vi "Process input and Make Stacks.vi"(11 "input":string[](array[string])) -> (2 "Moves":string[](array[string]), 3 "Stacks":cluster{"Label":string, "Stack":string[]}[](array[cluster]))   [LabVIEW 2021]
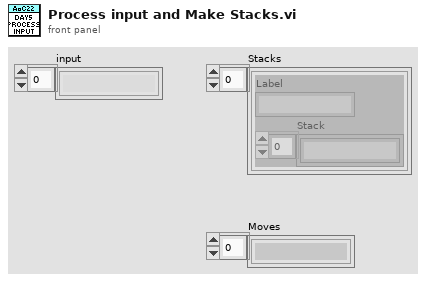
[diagram p1: front panel]
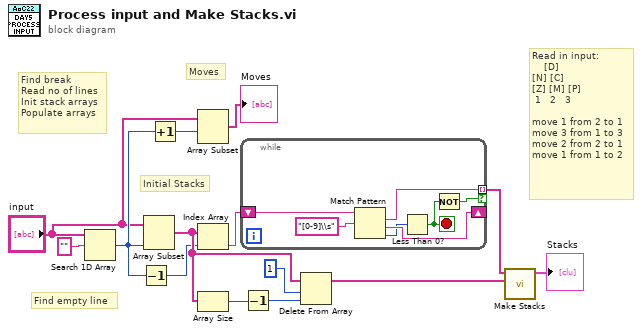
[diagram p0: block diagram]
diagram:
  # "Initial Stacks"
  # "Moves"
  # "Find empty line"
  # "Find break\nRead no of lines\nInit stack arrays\nPopulate arrays"
  # "Read in input:\n    [D]    \n[N] [C]    \n[Z] [M] [P]\n 1   2   3 \n\nmove 1 from 2 to 1\nmove 3 from 1 to 3\nmove 2 from 2 to 1\nmove 1 from 1 to 2"
  n1 = Search 1D Array(1D array="input", element="") -> (index of element=w11:i32)  [unwired: 1 in]
  n2 = Decrement(x=w11) -> (x-1=w5:i32)
  n3 = Array Subset(array="input", length=w11) -> (w6:string[])  [unwired: 1 in]
  n4 = Increment(x=w11) -> (x+1=w12:i32)
  n5 = Array Subset(array="input", index=w12) -> (→"Moves":string[])  [unwired: 1 in]
  n6 = Index Array(array=w6, index=w5) -> (element=w13:string)
  n7 = Array Size(array=w6) -> (size(s)=w7:i32)
  n8 = while {
    shift-right: [w19] -> _
    shift-left: w13 -> [w21]
    tunnel: [w18] -> w2 mode=indexing if=w15
    stop <- w16 stop-if-true
    n9 = Match Pattern(string=w21, regular expression="[0-9]\\s") -> (match substring=w18:string, after substring=w19:string, offset past match=w17:i32)  [unwired: 1 in, 1 out]
    n10 = Less Than 0?(x=w17) -> (x < 0?=w16:bool)
    n11 = Not(x=w16) -> (.not. x?=w15:bool)
  }
  n12 = Decrement(x=w7) -> (x-1=w8:i32)
  n13 = Delete From Array(array=w6, length=1, index=w8) -> (array with subset deleted=w3:string[])  [unwired: 1 out]
  n14 = call "Make Stacks.vi"("Stacks in"=w3, "Labels"=w2) -> ("Stacks out"=→"Stacks":cluster{"Label":string, "Stack":string[]}[])  [unwired: 9 in]
